vi "trace_denoise.vi"(0 "filter type":i32, 1 "filter":bool, 2 "Trace (r=wl, c=d)":dbl[][](array[numeric])) -> (6 "Denoised trace":dbl[][](array[numeric]))   [LabVIEW 2022 SP3]
uses:
  <vilib>/Analysis/3filter.llb/Filter Passband Type.ctl
  <vilib>/Analysis/3filter.llb/Chebyshev Filter (DBL).vi
  <vilib>/Analysis/3filter.llb/Butterworth Filter (DBL).vi
  <vilib>/Analysis/NI_AALBase.lvlib
panel:
  out "lowpass chebyshev":dbl[][](graph)
  out "lowpass butterworth":dbl[][](graph)
  out "raw":dbl[][](graph)
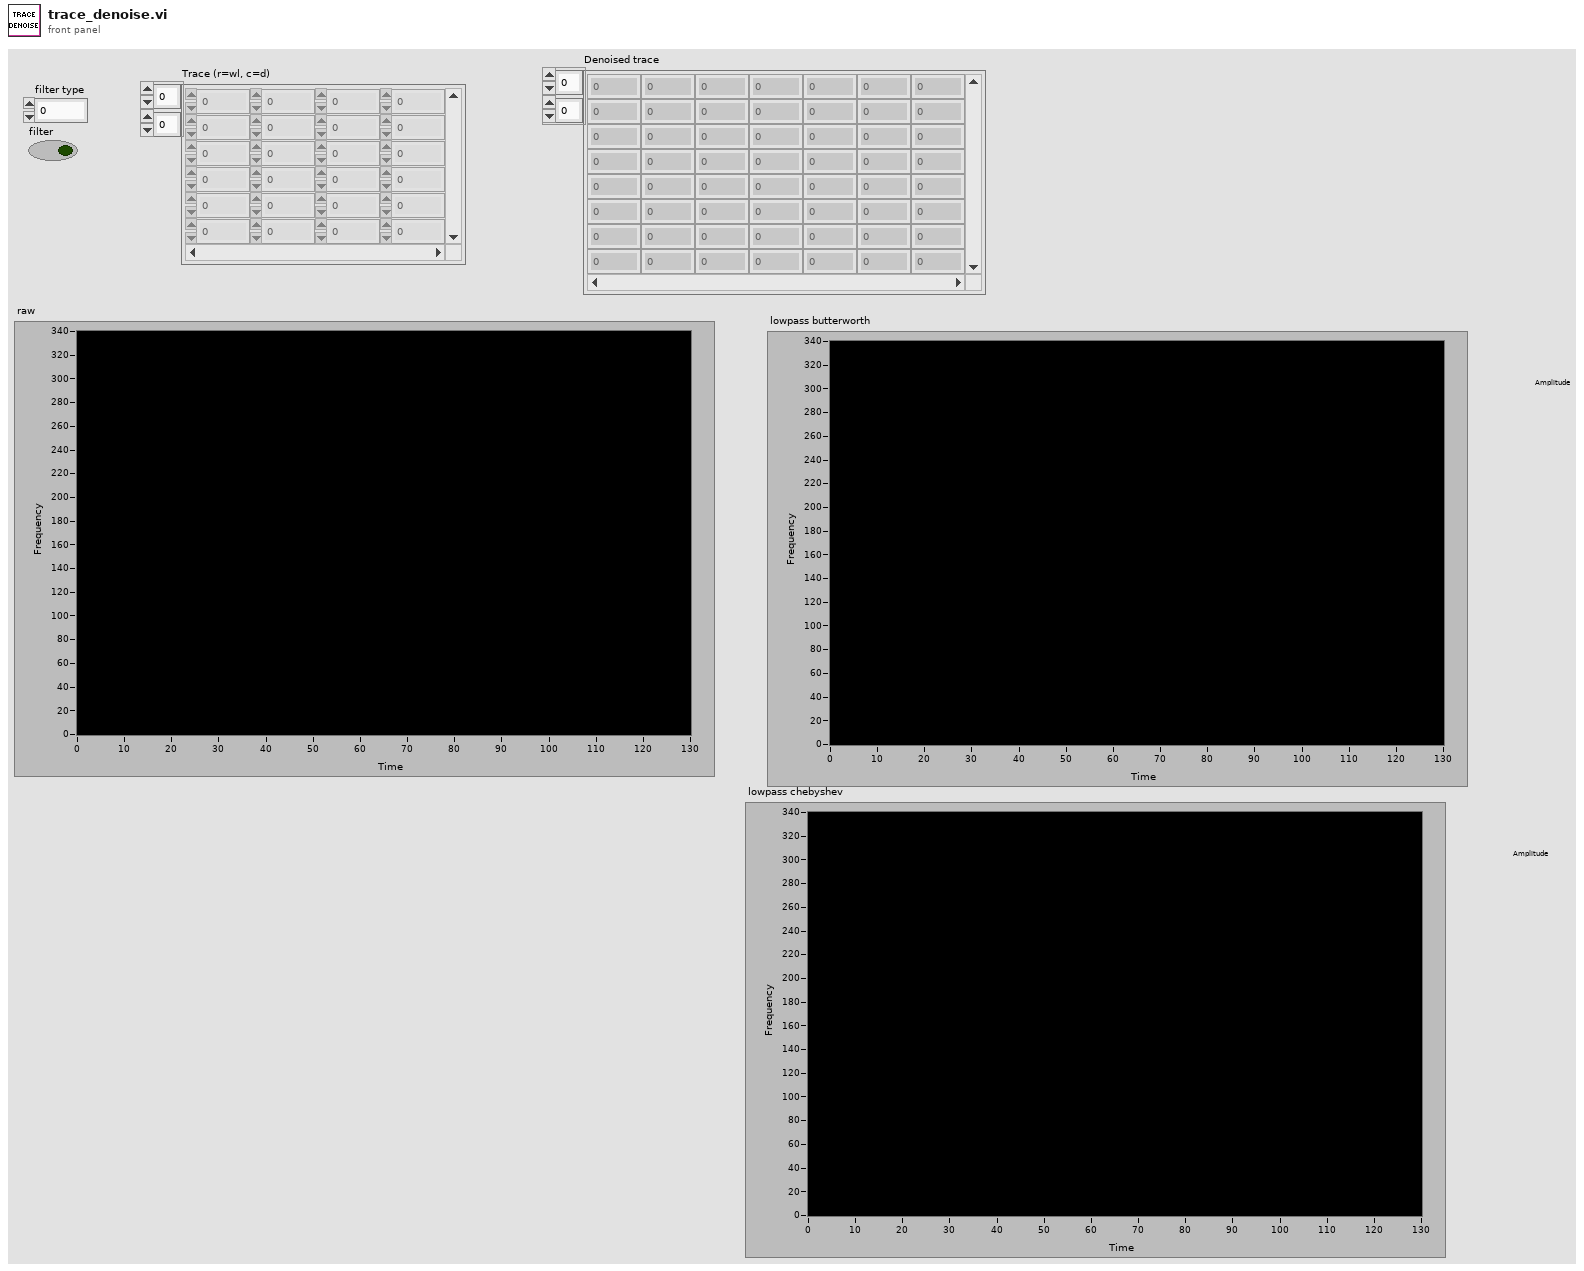
[diagram p1: front panel]
types:
  T1 = typedef "NI_AALBase.lvlib/Filter Passband Type.ctl" = enum32{"Lowpass", "Highpass", "Bandpass", "Bandstop"}
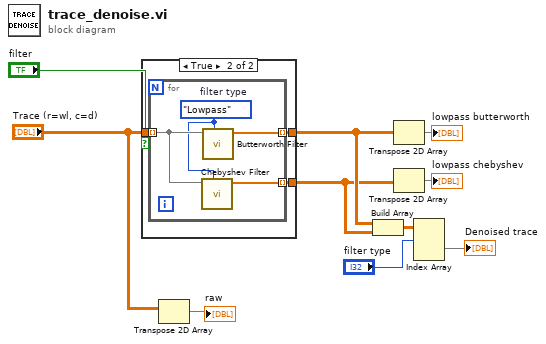
[diagram p0: block diagram]
diagram:
  n1 = case shown="True" "filter" {
    tunnel: "Trace (r=wl, c=d)" -> [w11 w14]
    tunnel: [w11 w13] -> w5
    tunnel: [w11 w12] -> w6
    frame False {
    }
    frame True {
      n2 = for {
        tunnel: w14 -> [w17] mode=indexing
        tunnel: [w18] -> w12 mode=indexing
        tunnel: [w15] -> w13 mode=indexing
        w16 = Filter_Passband_Type."Lowpass"  # filter type
        n3 = call-poly <vilib>:"Chebyshev Filter.vi"("filter type"=w16, "X"=w17) -> ("Filtered X"=w15:dbl[])  [unwired: 8 in, 1 out]
        n4 = call-poly <vilib>:"Butterworth Filter.vi"("filter type"=w16, "X"=w17) -> ("Filtered X"=w18:dbl[])  [unwired: 6 in, 1 out]
      }
    }
  }
  n5 = Transpose 2D Array(2D array="Trace (r=wl, c=d)") -> (transposed array=→"raw":dbl[][])
  n6 = Build Array(w6, w5) -> (w4:dbl[][][])
  n7 = Transpose 2D Array(2D array=w6) -> (transposed array=→"lowpass butterworth":dbl[][])
  n8 = Transpose 2D Array(2D array=w5) -> (transposed array=→"lowpass chebyshev":dbl[][])
  n9 = Index Array(array=w4, index (dim 0)="filter type") -> (element=→"Denoised trace":dbl[][])  [unwired: 2 in]
